vi "Has Next.vi"(8 "error in (no error)":errorcluster, 11 "Continuous.lvclass in":refnum<class "Continuous.lvclass">) -> (0 "error out":errorcluster, 2 "Again?":bool, 3 "Continuous.lvclass out":refnum<class "Continuous.lvclass">)   [LabVIEW 2017, in "Continuous.lvclass"]
uses:
  Continuous.lvclass
  Instruments/Oxford Magnet/Power Supply/Power Supply.lvclass
  C:/LabVIEW-programs/Instruments/Utility Classes/Scannable/Scannable.lvclass
  Scanner/Scanner.lvclass
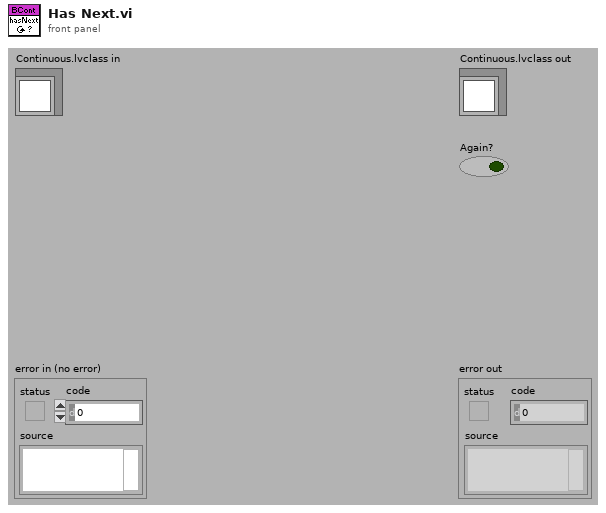
[diagram p1: front panel]
types:
  T1 = typedef "Scanner.lvclass/Range.ctl" = cluster{"xi":dbl, "xf":dbl, "dx":dbl, "Return to...?":bool, "Return to":dbl}
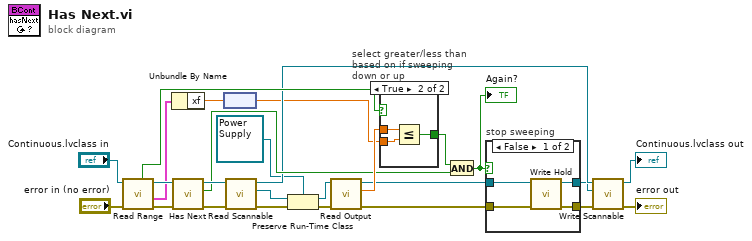
[diagram p0: block diagram]
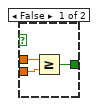
[diagram p2: hidden frame]
diagram:
  n1 = call-dynamic "Read Range.vi"("error in (no error)"="error in (no error)", "Scanner.lvclass in"="Continuous.lvclass in") -> ("error out"=w18:errorcluster, "Range"=w1:T1, "Scanner.lvclass out"=w25:refnum<class "Continuous.lvclass">, "Scanning Up?"=w17:bool)  [unwired: 6 out]
  n2 = Unbundle By Name(w1) -> ("xf"=w16:dbl)
  n3 = call-parent "Has Next.vi"("error in (no error)"=w18, "Scanner.lvclass in"=w25) -> ("error out"=w7:errorcluster, "Again?"=w21:bool, "Scanner.lvclass out"=w23:refnum<class "Continuous.lvclass">)  [unwired: 7 out]
  n4 = node(w16) -> (w2:dbl[unit])
  n5 = call-dynamic "Read Scannable.vi"("error in (no error)"=w7, "Scanner.lvclass in"=w23) -> ("error out"=w8:errorcluster, "Scannable.lvclass"=w12:refnum<class "Scannable.lvclass">, "Scanner.lvclass out"=w14:refnum<class "Continuous.lvclass">)  [unwired: 7 in]
  n6 = Preserve Run-Time Class(object in=w12, error in=w8, 2:refnum<class "Power Supply.lvclass"> refnum ("Power Supply out")) -> (object out=w10:refnum<class "Power Supply.lvclass">, error out=w9:errorcluster)
  n7 = call-dynamic "Read Output.vi"("error in (no error)"=w9, "Power Supply in"=w10) -> ("error out"=w4:errorcluster, "Field"=w24:dbl[unit], "Power Supply out"=w15:refnum<class "Power Supply.lvclass">)  [unwired: 5 in, 2 out]
  n8 = case "select greater/less than based on if sweeping down or up" shown="True" w17 {
    tunnel: w24 -> [w29 w32]
    tunnel: w2 -> [w28 w30]
    tunnel: [w27 w31] -> w22
    frame False {
      n9 = Greater Or Equal?(x=w29, y=w28) -> (x >= y?=w27:bool)
    }
    frame True {
      n10 = Less Or Equal?(x=w32, y=w30) -> (x <= y?=w31:bool)
    }
  }
  n11 = And(x=w22, y=w21) -> (x .and. y?=w20:bool)
  "Again?" <- w20
  n12 = case "stop sweeping" shown="False" w20 {
    tunnel: w15 -> [w36 w38]
    tunnel: [w35 w37] -> w5
    tunnel: w4 -> [w34 w37]
    tunnel: [w33 w38] -> w3
    frame False {
      n13 = call-dynamic "Write Hold.vi"("error in (no error)"=w34, "Power Supply in"=w36) -> ("error out"=w35:errorcluster, "Power Supply out"=w33:refnum<class "Power Supply.lvclass">)  [unwired: 8 in]
    }
    frame True {
    }
  }
  n14 = call-dynamic "Write Scannable.vi"("error in (no error)"=w5, "Scannable.lvclass"=w3, "Scanner.lvclass in"=w14) -> ("error out"=→"error out":errorcluster, "Scanner.lvclass out"=→"Continuous.lvclass out":refnum<class "Continuous.lvclass">)  [unwired: 7 in]
